vi "crop_image_to_SLM_size.vi"(6 "Y max":u16, 7 "X max":u16, 8 "error in (no error)":errorcluster, 9 "Y size":u16, 10 "X size":u16, 11 "Image Src":T1) -> (0 "error out":errorcluster, 3 "Image Dst Out":T1)   [LabVIEW 2025]
uses:
  <vilib>/vision/Image Controls.llb/IMAQ Image.ctl
  <vilib>/vision/NI_Vision_Development_Module.lvlib
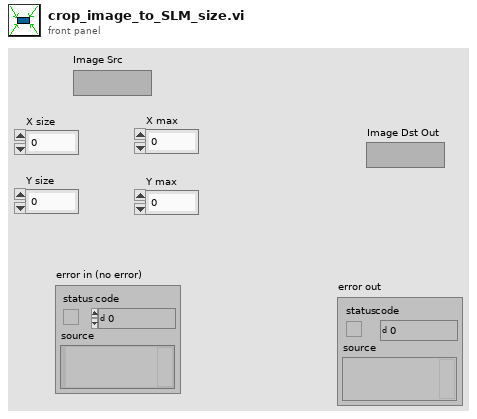
[diagram p1: front panel]
types:
  T1 = typedef "IMAQ Image.ctl" = refnum<image>
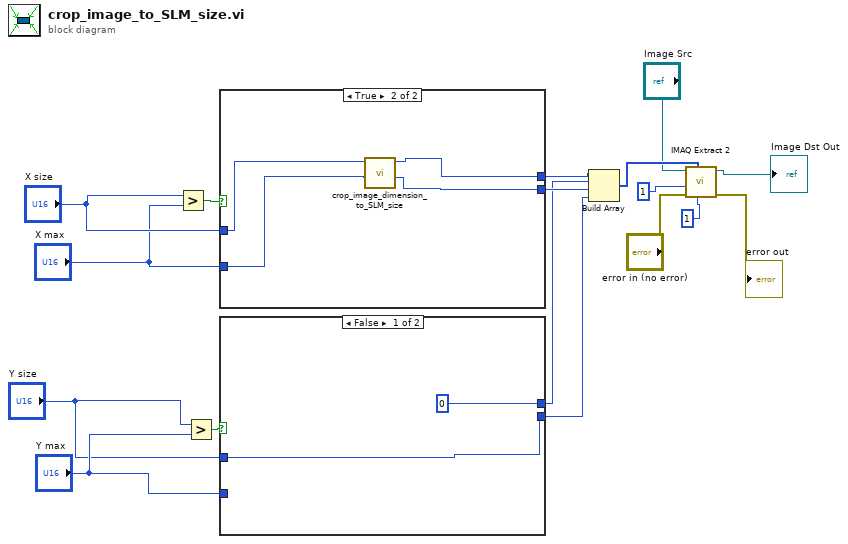
[diagram p0: block diagram]
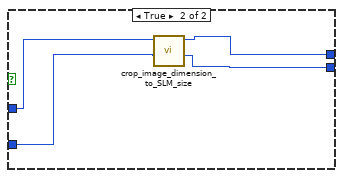
[diagram p2: hidden frame]
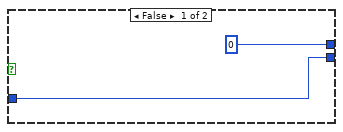
[diagram p3: hidden frame]
diagram:
  n1 = Greater?(x="X size", y="X max") -> (0:w17:bool)
  n2 = Greater?(x="Y size", y="Y max") -> (0:w8:bool)
  n3 = case shown="True" w17 {
    tunnel: [u16 0 w23] -> w12
    tunnel: [w18 w22] -> w11
    tunnel: "X size" -> [w18 w21]
    tunnel: "X max" -> [_ w20]
    frame False {
    }
    frame True {
      n4 = call "crop_image_dimension_to_SLM_size.vi"("max size"=w20, "original size"=w21) -> ("end index"=w22:u16, "start index"=w23:u16)  [unwired: 8 in]
    }
  }
  n5 = case shown="False" w8 {
    tunnel: [u16 0 w29] -> w5
    tunnel: [w24 w28] -> w4
    tunnel: "Y size" -> [w24 w27]
    tunnel: "Y max" -> [_ w26]
    frame False {
    }
    frame True {
      n6 = call "crop_image_dimension_to_SLM_size.vi"("max size"=w26, "original size"=w27) -> ("end index"=w28:u16, "start index"=w29:u16)  [unwired: 8 in]
    }
  }
  n7 = Build Array(w12, w5, w11, w4) -> (w14:u16[])
  n8 = call "IMAQ Extract 2"("Y Step Size"=1, "Optional Rectangle"=w14, "error in (no error)"="error in (no error)", "X Step Size"=1, "Image Src"="Image Src") -> ("error out"=→"error out":errorcluster, "Image Dst Out"=→"Image Dst Out":T1)  [unwired: 5 in]
